vi "OC2 Read Alarms.vi"(3 "error in (no error)":errorcluster, 4 "alarm report in":T1 {"Temp limt Max" format="%.1f"; "Temp limt Min" format="%.1f"; "Temp ok max" format="%.2f"; "Temp ok min" format="%.2f"; "Alarm Max" format="%.2f"; "Alarm Min" format="%.2f"; "Alarms" items=["Off", "Min", "Max", "Both"]}, 5 "enable":bool, 6 "VISA resource name":refnum<visa-resource-name>) -> (0 "error out":errorcluster, 1 "alarm report out":T1 {"Temp limt Max" format="%.1f"; "Temp limt Min" format="%.1f"; "Temp ok max" format="%.2f"; "Temp ok min" format="%.2f"; "Alarm Max" format="%.2f"; "Alarm Min" format="%.2f"; "Alarms" items=["Off", "Min", "Max", "Both"]}, 2 "dup VISA resource name":refnum<visa-resource-name>)   [LabVIEW 2009]
doc: "TCM Read Alarm.vi\n\nVI that reads the alarm information, accepts a cluster that contains the following variables:\nAlarms - of, min, max and both, reads which alarms are enabled\nAlarm min - minimum alarm temperature\nAlarm Max - maximum alarm value\nTemp ok min - \nTemp ok max - \nTemp limit min -\nTemp limit max -\n\nCOPYRIGHT ELECTRON DYNAMICS LTD"
panel:
  in  "Command":string
  out "Rx string":string
  # "Read Alarm"
  # "V1.02"
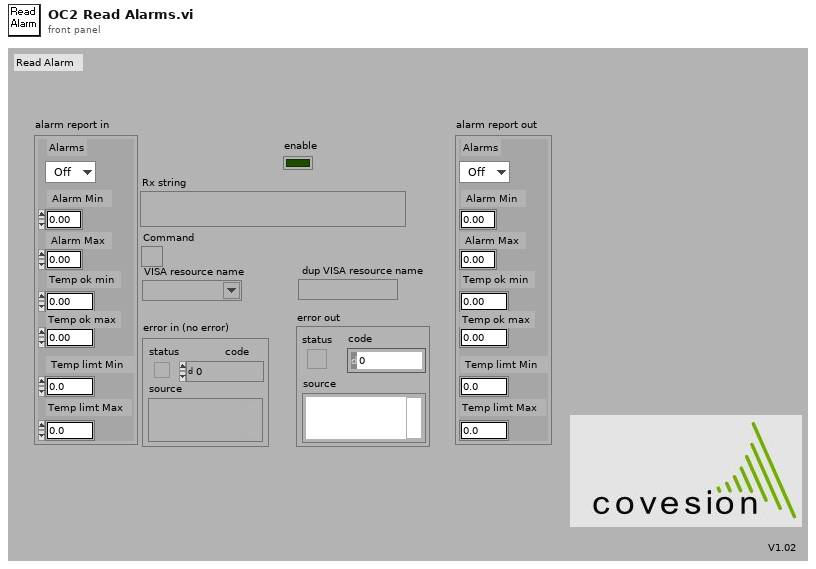
[diagram p1: front panel]
types:
  T1 = cluster{"Alarms":u16, " Alarm Min ":dbl, " Alarm Max ":dbl, "Temp ok min":dbl, "Temp ok max":dbl, " Temp limt Min ":dbl, "Temp limt Max ":dbl}
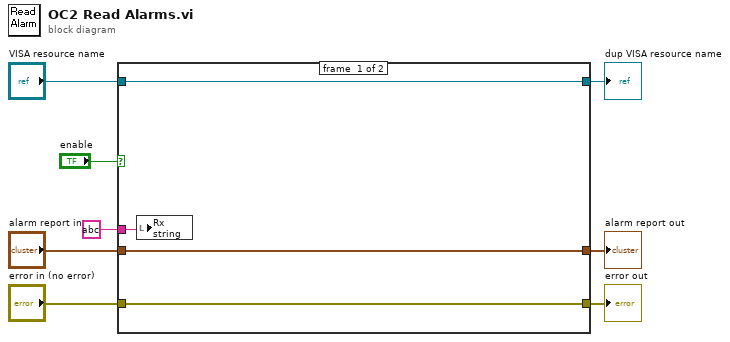
[diagram p0: block diagram]
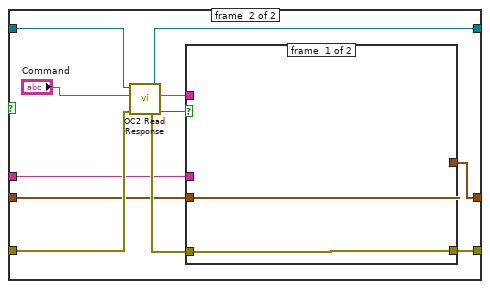
[diagram p2: hidden frame]
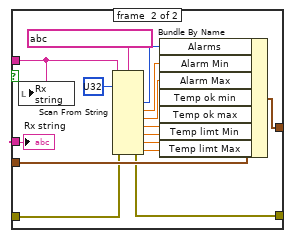
[diagram p3: hidden frame]
diagram:
  n1 = case shown="True" "enable" {
    tunnel: "VISA resource name" -> [w12 w20]
    tunnel: "error in (no error)" -> [w10 w19]
    tunnel: [w12 w17] -> w6
    tunnel: "alarm report in" -> [w11 w16]
    tunnel: [w10 w15] -> w4
    tunnel: [w11 w14] -> w3
    tunnel: string ? ("Rx string") -> [w9 w13]
    frame #0 {
      n2 = local write "Rx string"(w9) -> ()
    }
    frame #1 {
      n3 = call "OC2 Read Response.vi"("error in (no error)"=w19, "Command"="Command", "VISA resource name"=w20) -> ("RX packet ok"=w21:bool, "error out"=w18:errorcluster, "output string"=w23:string, "dup VISA resource name"=w17:refnum<visa-resource-name>)  [unwired: 1 in]
      n4 = case shown="True" w21 {
        tunnel: w23 -> [_ w38]
        tunnel: w18 -> [w24 w29]
        tunnel: w16 -> [w25 w37]
        tunnel: [w24 w28] -> w15
        tunnel: [w25 w27] -> w14
        tunnel: w13 -> [_ w26]
        frame #0 {
        }
        frame #1 {
          n5 = local write "Rx string"(w38) -> ()
          n6 = Scan From String(format string=string ?, input string=w38, initial scan location=u32 ?, error in=w29) -> (error out=w28:errorcluster, output 1=w30:i32, output 2=w31:dbl, output 3=w32:dbl, output 4=w33:dbl, output 5=w34:dbl, output 6=w35:dbl, output 7=w36:dbl)  [unwired: 7 in, 2 out]
          n7 = Bundle By Name(cluster=w37, "Alarms"=w30, "Alarm Min"=w31, "Alarm Max"=w32, "Temp ok min"=w33, "Temp ok max"=w34, "Temp limt Min"=w35, "Temp limt Max"=w36) -> (w27:T1)
          "Rx string" <- w26
        }
      }
    }
  }
  "error out" <- w4
  "dup VISA resource name" <- w6
  "alarm report out" <- w3
